vi "ma_Extract multiple tones info from spectrum.vi"(7 "spectrum includes end points?":bool, 8 "error in":errorcluster, 9 "criterion":T1={"Single/Multiple"=enum."Multiple Peaks", "Threshold"=0.0, "max #tones"=4} {"Threshold" format="%.2f"}, 10 "spectral info":T3 {"window" items=["Rectangle"=0, "Hanning"=1, "Hamming"=2, "Blackman-Harris"=3, "Exact Blackman"=4, "Blackman"=5, "Flat Top"=6, "4 Term B-Harris "=7, "7 Term B-Harris"=8, "Low Sidelobe"=9, "Blackman Nuttall"=11, "Triangle"=30, "Bartlett-Hanning"=31, "Bohman"=32, "Parzen"=33, "Welch"=34, "Kaiser"=60, "Dolph-Chebyshev"=61, "Gaussian"=62]}, 11 "FFT spectrum":cluster{"f0":dbl, "df":dbl, "spectrum":cdb[]}={"f0"=0.0, "df"=1.0, "spectrum"=[]} {"spectrum" format="%.2f"; "df" format="%.2f"; "f0" format="%.2f"}) -> (0 "error out":errorcluster, 2 "#tones":i32, 3 "extracted tones (sorted by amplitude)":T2(array[cluster]) {"phase [degree]" format="%.2f"; "amplitude" format="%.4f"; "frequency [Hz]" format="%.2f"})   [LabVIEW 2020, in "NI_MAPro.lvlib"]
uses:
  NI_MAPro.lvlib
  ma_sml_Spectral Info.ctl
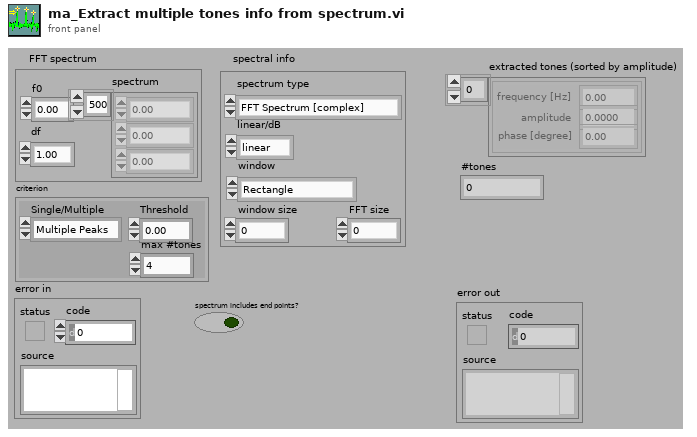
[diagram p1: front panel]
types:
  T1 = cluster{"Single/Multiple":enum16{"Multiple Peaks", "Single Max Peak"}, "Threshold":dbl, "max #tones":i32}
  T2 = cluster{"frequency [Hz]":dbl, "amplitude":dbl, "phase [degree]":dbl}[]
  T3 = typedef "NI_MAPro.lvlib/ma_sml_Spectral Info.ctl" = cluster{"spectrum type":enum16{"FFT Spectrum [complex]", "Amplitude [Magnitude]", "Power [Magnitude^2]", "Cross Spectrum [complex]", "Frequency Response [Complex]"}, "linear/dB":enum16{"linear", "dB"}, "window":u16, "window size":i32, "FFT size":i32}
  T4 = cluster{"frequency [Hz]":dbl, "amplitude":dbl, "phase [degree]":dbl}
  T5 = cluster{"Single/Multiple":enum16{"Multiple Peaks", "Single Max Peak"}, "Threshold":dbl}
  T6 = typedef "NI_MAPro.lvlib/ma_sml_Spectrum Cluster (complex).ctl" = cluster{"f0":dbl, "df":dbl, "spectrum":cdb[]}
  T7 = cluster{"frequency":dbl, "amplitude":dbl, "phase [degree]":dbl}
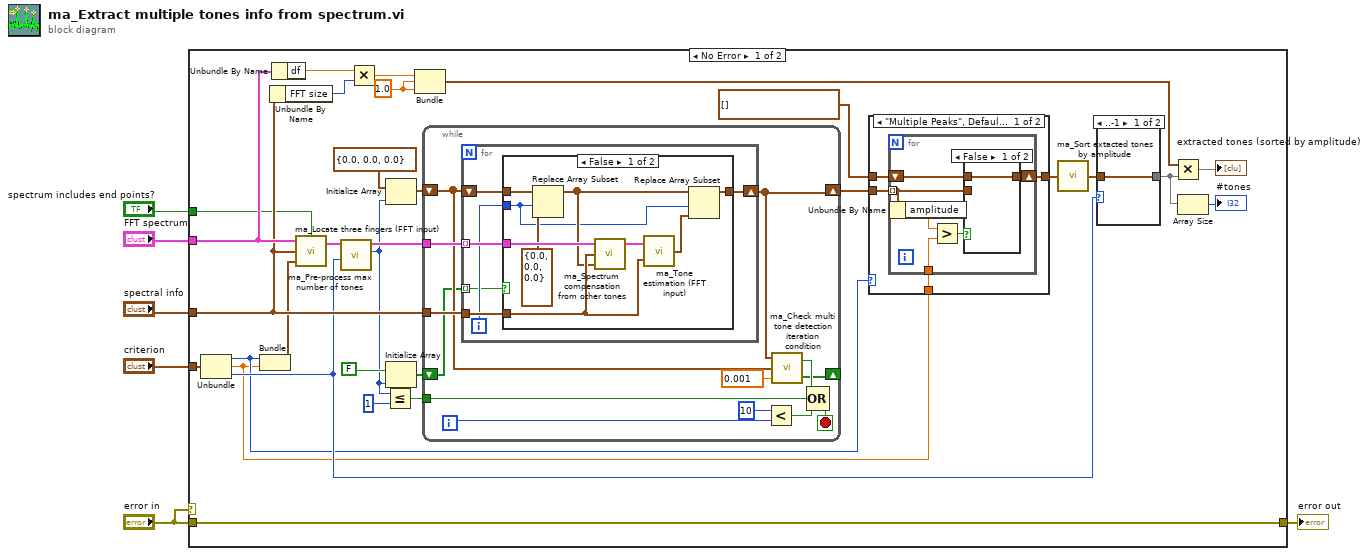
[diagram p0: block diagram]
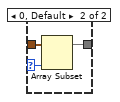
[diagram p2: hidden frame]
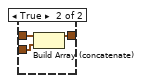
[diagram p4: hidden frame]
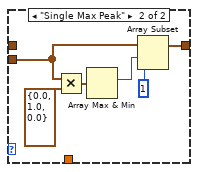
[diagram p5: hidden frame]
diagram:
  n1 = case shown="No Error" "error in" {
    tunnel: "error in" -> [w36 w90]
    tunnel: [w36 w90] -> w5
    tunnel: "spectral info" -> [w29 _]
    tunnel: "criterion" -> [w19 _]
    tunnel: "FFT spectrum" -> [w30 _]
    tunnel: "spectrum includes end points?" -> [w20 _]
    frame No Error {
      w8 = 1.0 ("x*y")
      n2 = Unbundle(w19) -> ("Single/Multiple"=w12:enum16{"Multiple Peaks", "Single Max Peak"}, "Threshold"=w9:dbl, "max #tones"=w14:i32)
      n3 = Bundle("Single/Multiple"=w12, "Threshold"=w9) -> (w18:T5)  [unwired: 1 out]
      n4 = Unbundle By Name(w29) -> ("FFT size"=w28:i32)
      n5 = Unbundle By Name(w30) -> ("df"=w27:dbl)
      n6 = call "ma_Locate three fingers (FFT input).vi"("spectrum includes end points?"=w20, "criterion"=w18, "spectral info"=w29, "FFT spectrum"=w30) -> ("three fingers (frequency normalized)"=w17:T6[])  [unwired: 1 out]
      n7 = call "ma_Pre-process max number of tones.vi"("max #tones"=w14, "three fingers in"=w17) -> ("number of tones"=w15:i32, "three fingers out"=w16:T6[])  [unwired: 8 out]
      n8 = Multiply(x=w27, y=w28) -> (x*y=w25:dbl)
      n9 = Less Or Equal?(x=w15, y=1) -> (x <= y?=w31:bool)
      n10 = Initialize Array(T4 {"frequency [Hz]"=0.0, "amplitude"=0.0, "phase [degree]"=0.0} ("single tone info."), w15) -> (w33:T2)
      n11 = Initialize Array(FALSE ("all stable?"), w15) -> (w22:bool[])
      n12 = Bundle(w25, "x*y"=w8, "x*y"=w8) -> (w26:cluster{dbl, "x*y":dbl, "x*y":dbl})  [unwired: 1 out]
      n13 = while {
        shift-left: w22 -> [w42]
        shift-right: [w41] -> _
        tunnel: w31 -> [w48]
        shift-left: w33 -> [w50]
        shift-right: [w51] -> w24
        tunnel: w29 -> [w52]
        tunnel: w16 -> [w53]
        i -> [w46]
        stop <- w44 stop-if-true
        n14 = for {
          tunnel: w53 -> [w58] mode=indexing
          shift-right: [w59] -> w51
          shift-left: w50 -> [w56]
          tunnel: w52 -> [w57]
          tunnel: w42 -> [w54] mode=indexing
          i -> [w55]
          n15 = case shown="False" w54 {
            tunnel: [w68 w69] -> w59
            tunnel: w58 -> [w67 _]
            tunnel: w57 -> [w66 _]
            tunnel: w56 -> [w64 w69]
            tunnel: w55 -> [w60 _]
            frame False {
              n16 = Replace Array Subset(array=w64, new element=T4 {"frequency [Hz]"=0.0, "amplitude"=0.0, "phase [degree]"=0.0} ("single tone info."), index=w60) -> (w62:T2)
              n17 = call "ma_Spectrum compensation from other tones.vi"("other tones' information"=w62, "spectral info"=w66, "FFT spectrum"=w67) -> ("compensated FFT spectrum"=w65:T6)
              n18 = call "ma_Tone estimation (FFT input).vi"("spectral info"=w66, "three fingers"=w65) -> ("single tone info."=w61:T7)
              n19 = Replace Array Subset(array=w62, new element=w61, index=w60) -> (w68:T2)
            }
            frame True {
            }
          }
        }
        n20 = Less?(x=10, y=w46) -> (x < y?=w47:bool)
        n21 = call "ma_Check multi tone detection iteration condition.vi"("precision"=0.001, "peaks before"=w50, "peaks after"=w51) -> ("stable?"=w41:bool[], "all stable?"=w49:bool)
        n22 = Compound Arithmetic op=OR(w49, w48, w47) -> (w44:bool)
      }
      n23 = case shown="\"Multiple Peaks\", Default" w12 {
        tunnel: w24 -> [w73 w87]
        tunnel: T2 [] ("Output Array") -> [w72 _]
        tunnel: w9 -> [w71 _]
        tunnel: [w70 w84] -> w11
        frame "Multiple Peaks", Default {
          n24 = for {
            tunnel: w73 -> [w75] mode=indexing
            shift-right: [w74] -> w70
            shift-left: w72 -> [w76]
            tunnel: w71 -> [w78]
            n25 = Unbundle By Name(w75) -> ("amplitude"=w79:dbl)
            n26 = Greater?(x=w79, y=w78) -> (0:w77:bool)
            n27 = case shown="False" w77 {
              tunnel: w76 -> [w80 w83]
              tunnel: w75 -> [_ w82]
              tunnel: [w80 w81] -> w74
              frame False {
              }
              frame True {
                n28 = Build Array (concatenate)(w83, w82) -> (w81:T2)
              }
            }
          }
        }
        frame "Single Max Peak" {
          n29 = Multiply(x=w87, y=T4 {"frequency [Hz]"=0.0, "amplitude"=1.0, "phase [degree]"=0.0} ("single tone info.")) -> (x*y=w88:T2)
          n30 = Array Max & Min(array=w88) -> (max index (indices)=w86:i32)  [unwired: 3 out]
          n31 = Array Subset(array=w87, index=w86, length=1 ("Array Length")) -> (w84:T2)
        }
      }
      n32 = call "ma_Sort extacted tones by amplitude.vi"("extracted tones in"=w11) -> ("extracted tones (sorted by amplitude)"=w10:T2)  [unwired: 4 out]
      n33 = case shown="..-1" w14 {
        selector: w14 -> [_ w38]
        tunnel: [w37 w39] -> w13
        tunnel: w10 -> [w37 w40]
        frame ..-1 {
        }
        frame 0, Default {
          n34 = Array Subset(array=w40, length=w38) -> (w39:T2)  [unwired: 1 in]
        }
      }
      n35 = Multiply(x=w26, y=w13) -> (x*y=→"extracted tones (sorted by amplitude)":cluster{dbl, dbl, dbl}[])
      n36 = Array Size(array=w13) -> (size(s)=→"#tones":i32)
    }
    frame Error {
    }
  }
  "error out" <- w5
